vi "Pot.Voltage to Angle_subVI.vi"(11 "Potentiometer V (0-5)":dbl) -> (3 "Pull-back angle (°)":dbl)   [LabVIEW 2017]
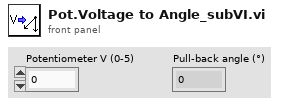
[diagram p1: front panel]
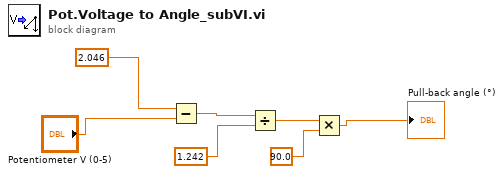
[diagram p0: block diagram]
diagram:
  n1 = Subtract(x=2.046, y="Potentiometer V (0-5)") -> (x-y=w3:dbl)
  n2 = Divide(x=w3, y=1.242) -> (x/y=w5:dbl)
  n3 = Multiply(x=w5, y=90.0) -> (x*y=→"Pull-back angle (°)":dbl)
